vi "GetResolution.vi"(8 "error in (no error)":errorcluster, 11 "CameraTestingProxyAPI in":refnum<class "CameraTestingProxyAPI.lvclass">) -> (0 "error out":errorcluster, 2 "Resolution":T1, 3 "CameraTestingProxyAPI out":refnum<class "CameraTestingProxyAPI.lvclass">)   [LabVIEW 2020, in "CameraTestingProxy.lvlib" / "CameraTestingProxyAPI.lvclass"]
uses:
  CameraTestingProxyAPI.lvclass
  381ef252-7ee6-412c-b175-a2d7afb6e14e.vi
  ICameraTestingProxy/TypeDef/Resolution.ctl
  ICameraTestingProxy/TypeDef/ICameraTestingProxy_typedef.lvlib
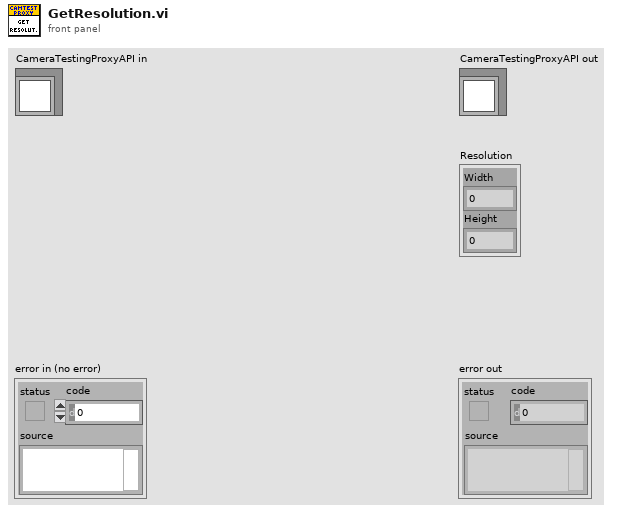
[diagram p1: front panel]
types:
  T1 = typedef "ICameraTestingProxy_typedef.lvlib/Resolution.ctl" = cluster{"Width":i16, "Height":i16}
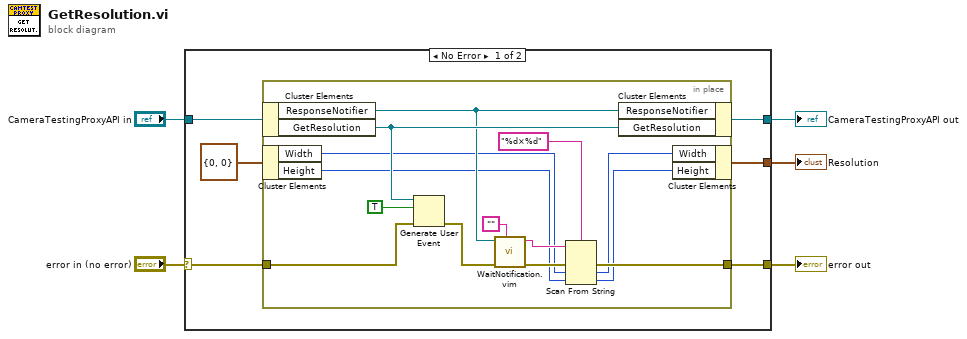
[diagram p0: block diagram]
diagram:
  n1 = case shown="No Error" "error in (no error)" {
    selector: "error in (no error)" -> [w9 w27]
    tunnel: "CameraTestingProxyAPI in" -> [w11 w26]
    tunnel: [w8 w27] -> w2
    tunnel: [w10 w26] -> w4
    tunnel: [w7 _] -> w1
    frame No Error {
      n2 = in-place {
        in-place-border: w9 -> [w25]
        in-place-border: [w19] -> w8
        n3 = in-place-cluster #1(w11) -> ("ResponseNotifier"=w21:refnum<notifier>, "GetResolution"=w22:refnum<user-event>)
        n4 = in-place-cluster #2(T1 {"Width"=0, "Height"=0} ("Resolution")) -> ("Width"=w16:i16, "Height"=w15:i16)
        n5 = Generate User Event(user event=w22, event data cluster=TRUE ("event data"), error in=w25) -> (error out=w24:errorcluster)  [unwired: 1 in, 1 out]
        n6 = call "WaitNotification.vim"("Type"="", "error in (no error)"=w24, "ResponseNotifier"=w21) -> ("error out"=w20:errorcluster, "Data"=w17:string)  [unwired: 7 in]
        n7 = Scan From String(format string="%d×%d", input string=w17, error in=w20, default 1=w16, default 2=w15) -> (error out=w19:errorcluster, output 1=w14:i16, output 2=w13:i16)  [unwired: 1 in, 2 out]
        n8 = in-place-cluster #1("ResponseNotifier"=w21, "GetResolution"=w22) -> (w10:refnum<class "CameraTestingProxyAPI.lvclass">)
        n9 = in-place-cluster #2("Width"=w14, "Height"=w13) -> (w7:T1)
      }
    }
    frame Error {
    }
  }
  "error out" <- w2
  "CameraTestingProxyAPI out" <- w4
  "Resolution" <- w1
